vi "Test My JKI State Machine API.vi"() -> ()   [LabVIEW 2017, in "CSM Example echo DQMH.lvlib"]
doc: "------------- lvcsm -------------\n[CSMStates]\nItem 0 = \"Event Structure\"\nItem 1 = \"Idle\"\nItem 2 = \"Critical Error\"\nItem 3 = \"Async Message Posted\"\nItem 4 = \"Target Timeout Error\"\nItem 5 = \"Target Error\"\nItem 6 = \"Async Response\"\nItem 7 = \"Response\"\nItem 8 = \"Initialize Core Data\"\nItem 9 = \"VI Reference\"\nItem 10 = \"Error Handler\"\nItem 11 = \"Exit\"\nItem 12 = \"Data: Initialize\"\nItem 13 = \"Data: Cleanup\"\nItem 14 = \"UI: Initialize\"\nItem 15 = \"UI: Cursor Set\"\nItem 16 = \"UI: Front Panel State\"\nItem 17 = \"Macro: Initialize\"\nItem 18 = \"Macro: Exit\"\nItem 19 = \"New Category: 1\"\nItem 20 = \"New Category: 2\"\nItem 21 = \"Module: Start Module\"\n\n[CSMStatus]"
uses:
  CSM Example echo DQMH.lvlib
  user.lib/_NEVSTOP/Communicable State Machine(CSM)/_Support/Common/Format Timestamp.vi
  user.lib/_NEVSTOP/Communicable State Machine(CSM)/_Polymophic/Build No-Reply Asynchronous Message with Arguments.vi
  user.lib/_NEVSTOP/Communicable State Machine(CSM)/Communicable State Machine.lvlib
panel:
  out "Active Module":string[](array[string])
  in  "Select  Module":string(combo)
  out "Reply":string
  in  "X":dbl=1.0
  in  "wait for reply":bool=TRUE
  out "Reply Payload":dbl
  in  "Stop Module":bool
  in  "Start Module":bool
  in  "Test Do Something Else and Wait for Reply":bool
  in  "Hide Module Panel":bool
  in  "Show Module Panel":bool
  in  "Test Do Something Else":bool
  in  "Test Do Something":bool
  # "1. Support both Singleton and Cloneable , compare with DQMH Template\n2. Use the reply method -> as the replacement of status report in DQMH Template"
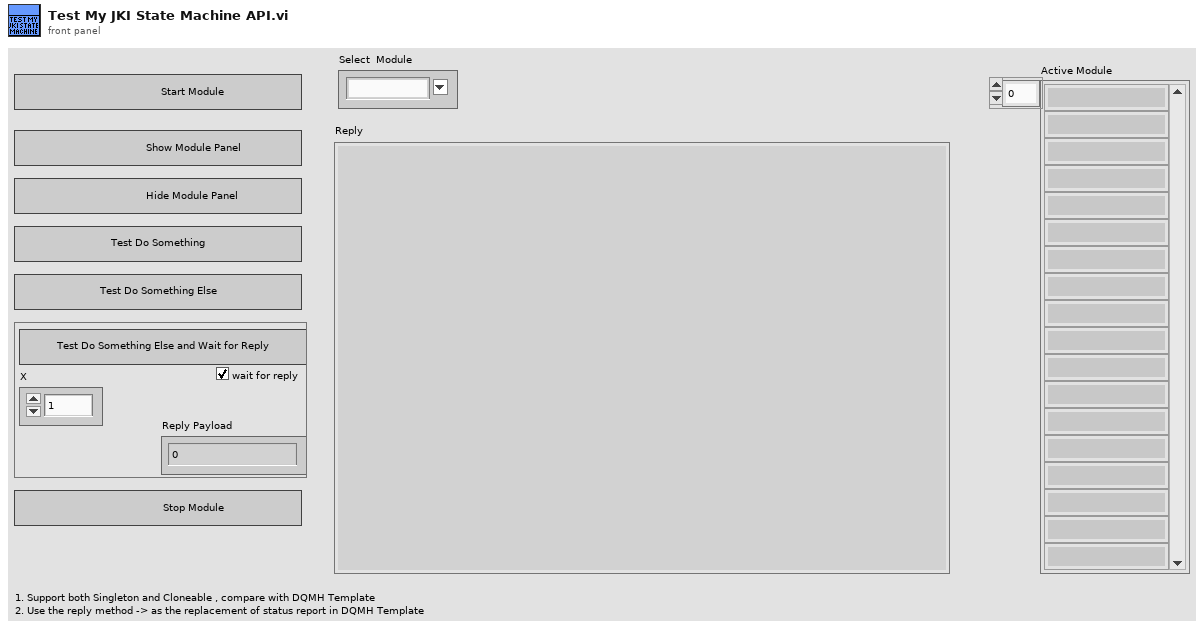
[diagram p1: front panel]
types:
  T1 = enum32{"Invalid", "Standard", "Closed", "Hidden", "Minimized", "Maximized"}
  T2 = enum32{"invalid app kind", "Development System", "Run Time System", "Student Edition", "Embedded LabVIEW", "Evaluation", "Custom"}
  T3 = typedef "Communicable State Machine.lvlib/_CSM_Response Source Message.ctl" = cluster{"‘State":string, "’Arguments":string, "’Error":errorcluster}
  T4 = cluster{"Core":cluster{"Current VI Reference":refnum<vi>, "Close Panel on Exit?":bool}, "Your Boolean data":bool, "Your string data":string, "Select  Module":refnum<vi>}
  T5 = cluster{"Current VI Reference":refnum<vi>, "Close Panel on Exit?":bool}
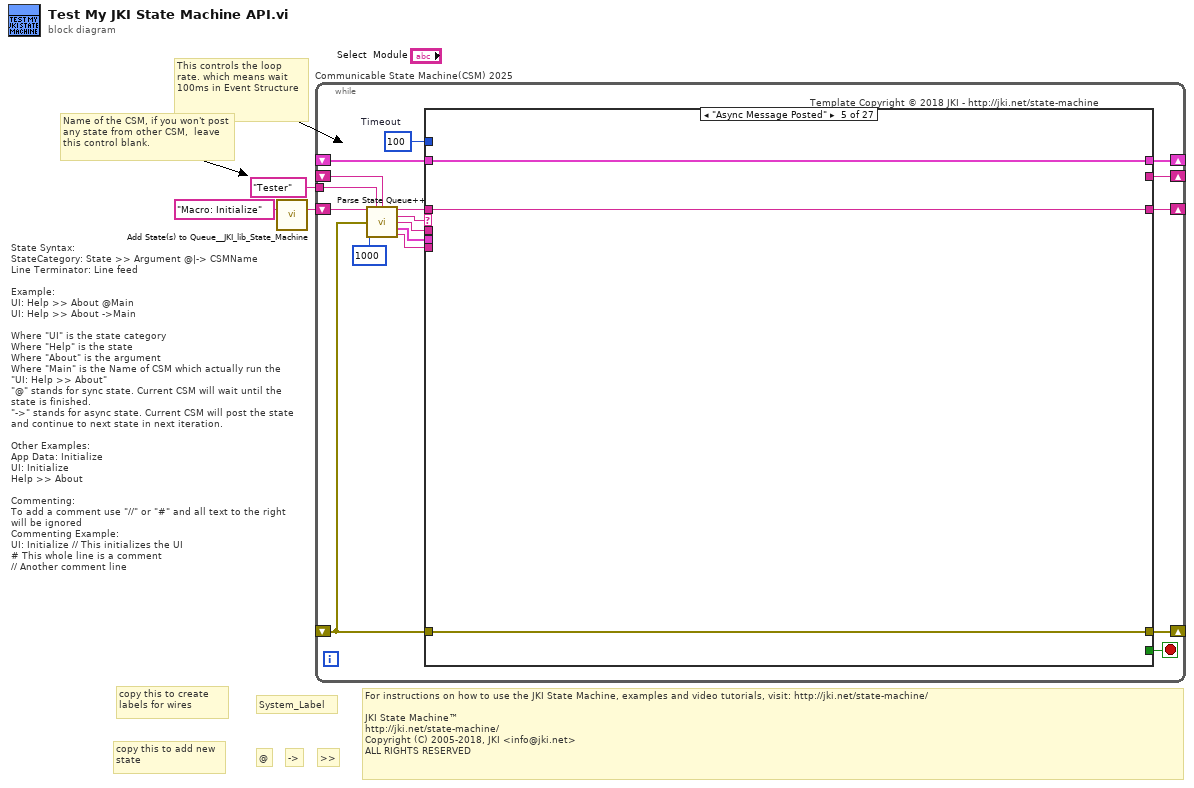
[diagram p0: block diagram]
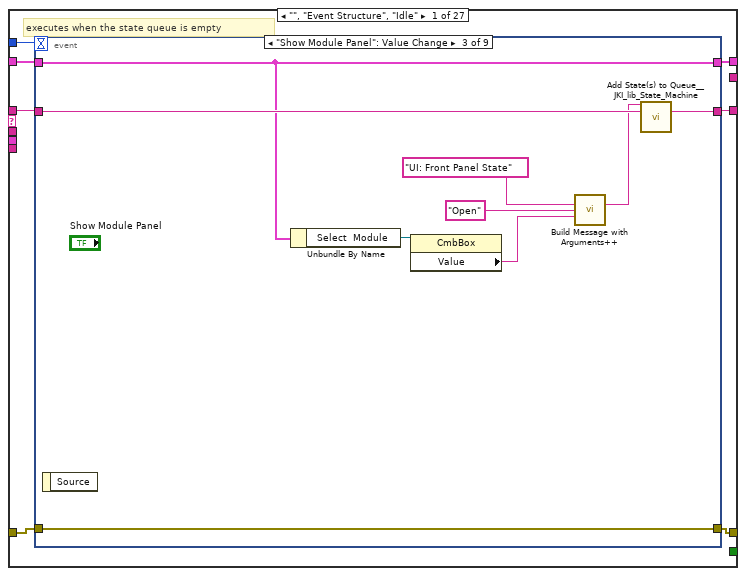
[diagram p2: hidden frame]
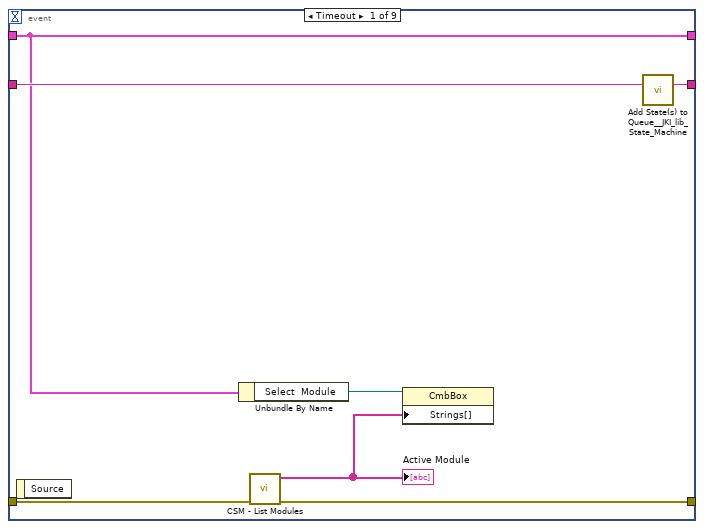
[diagram p3: hidden frame]
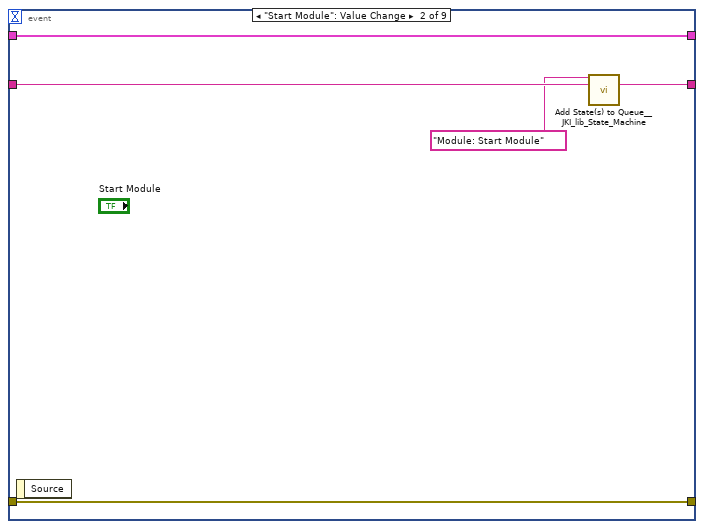
[diagram p4: hidden frame]
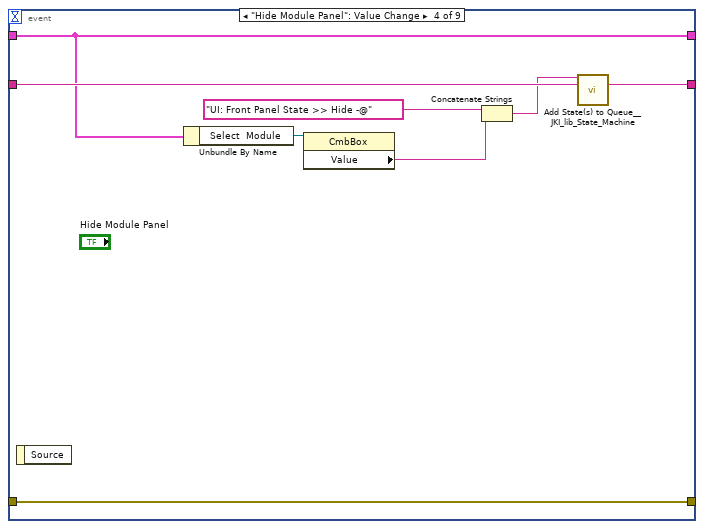
[diagram p5: hidden frame]
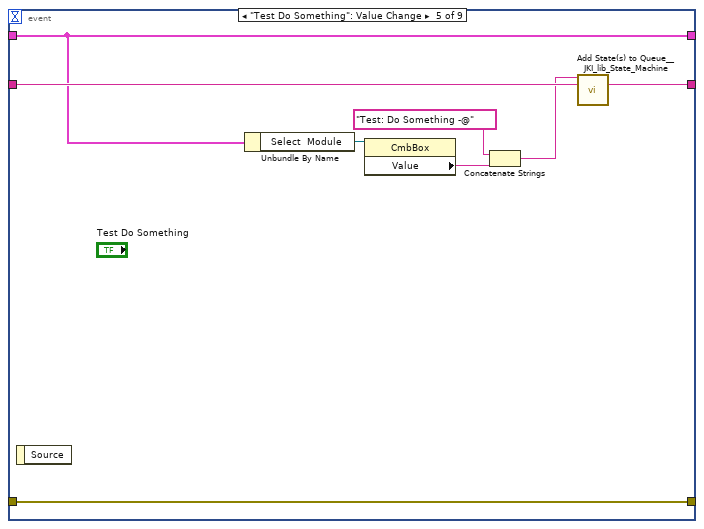
[diagram p6: hidden frame]
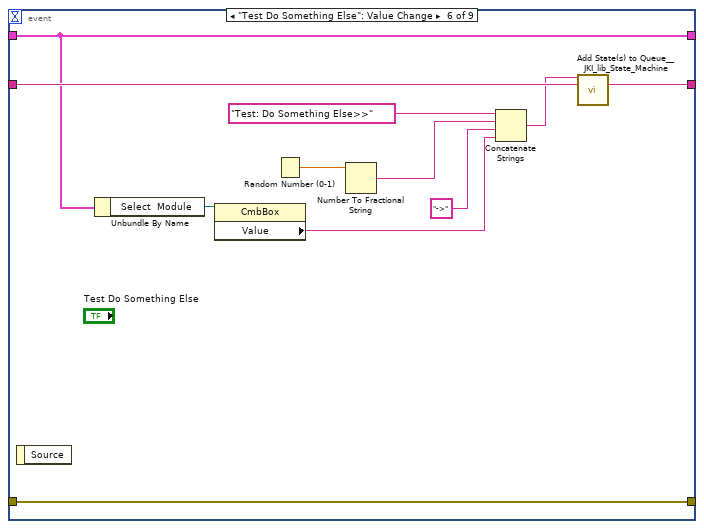
[diagram p7: hidden frame]
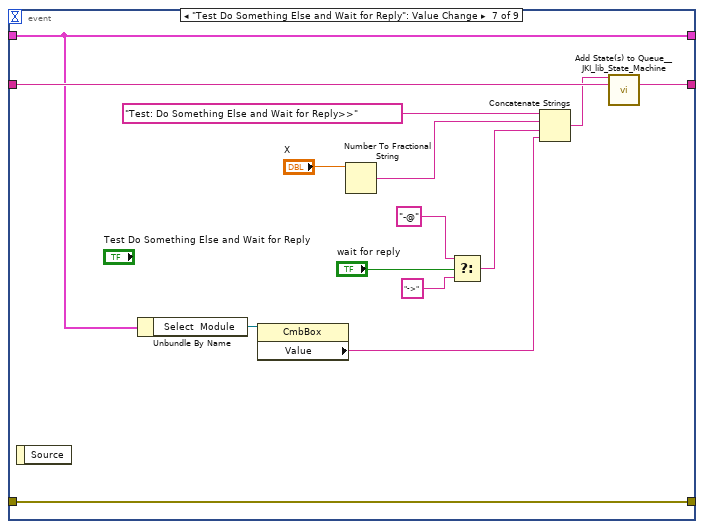
[diagram p8: hidden frame]
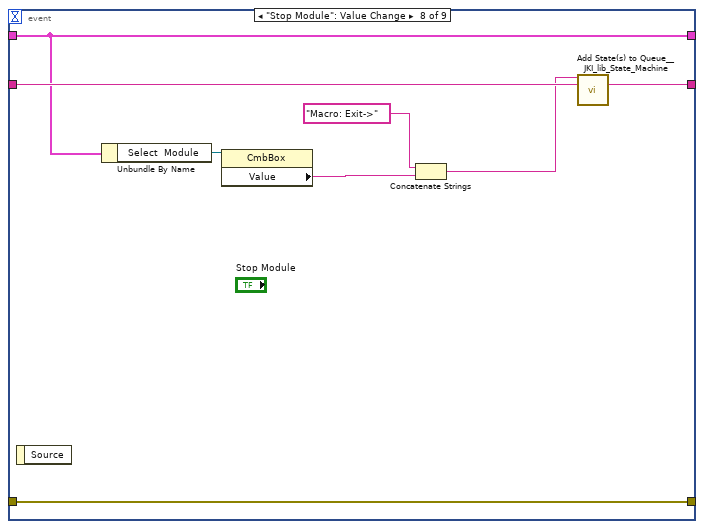
[diagram p9: hidden frame]
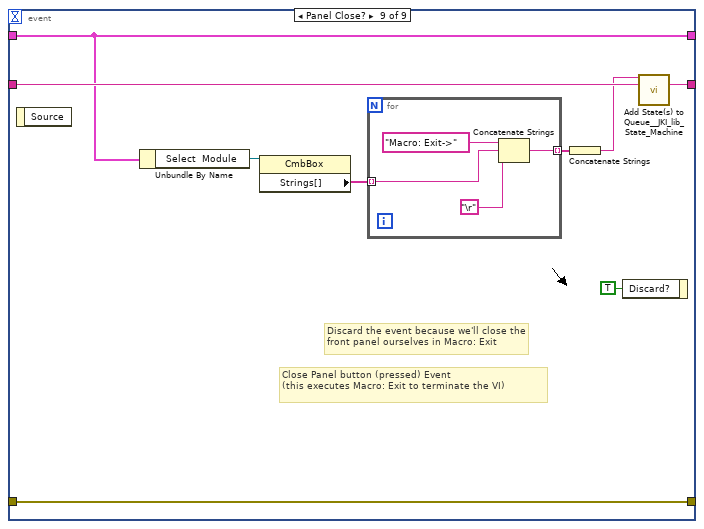
[diagram p10: hidden frame]
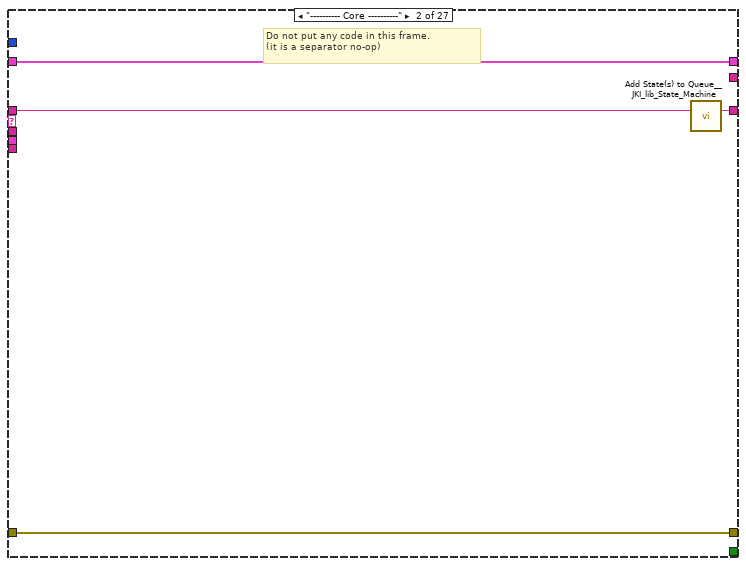
[diagram p11: hidden frame]
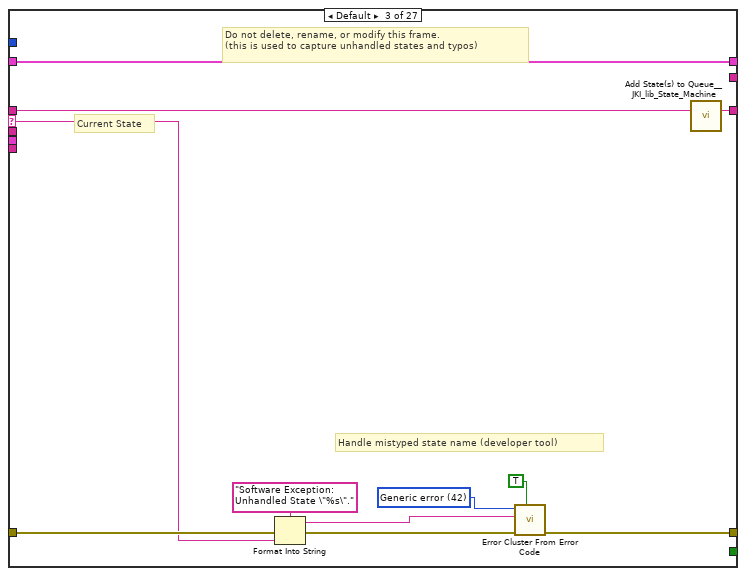
[diagram p12: hidden frame]
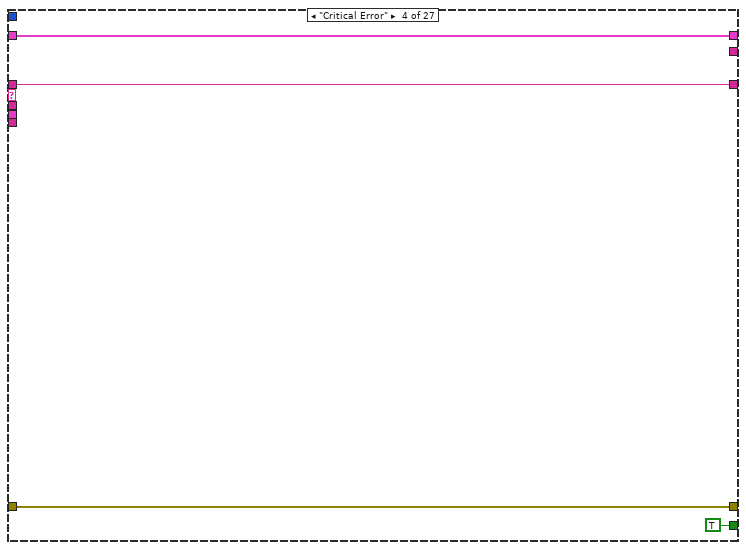
[diagram p13: hidden frame]
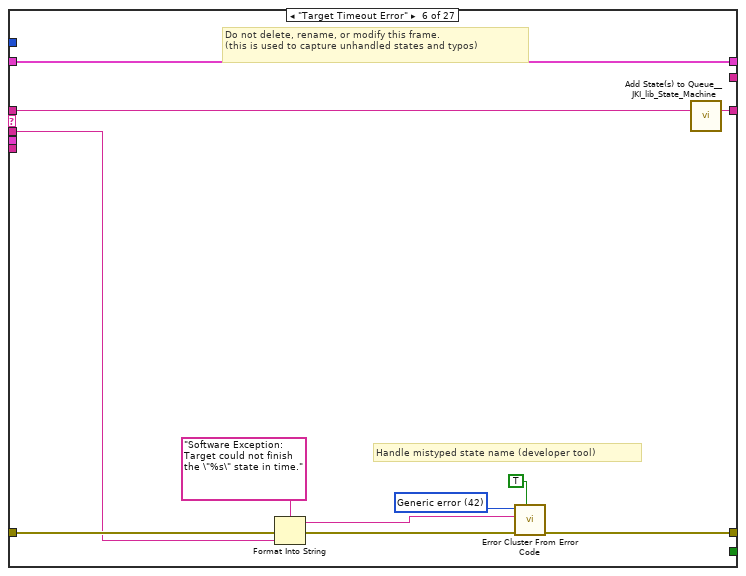
[diagram p14: hidden frame]
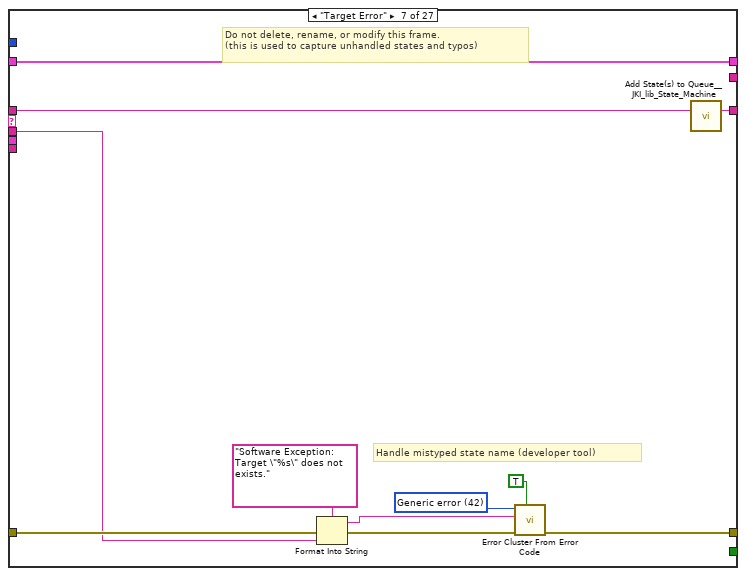
[diagram p15: hidden frame]
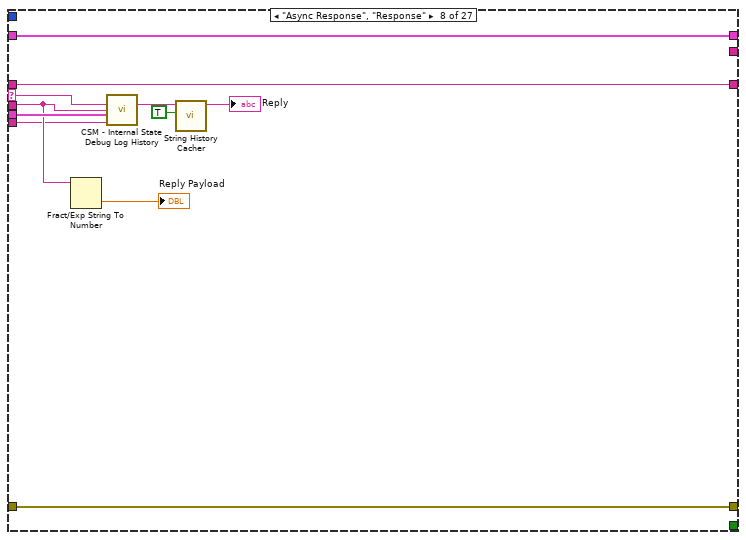
[diagram p16: hidden frame]
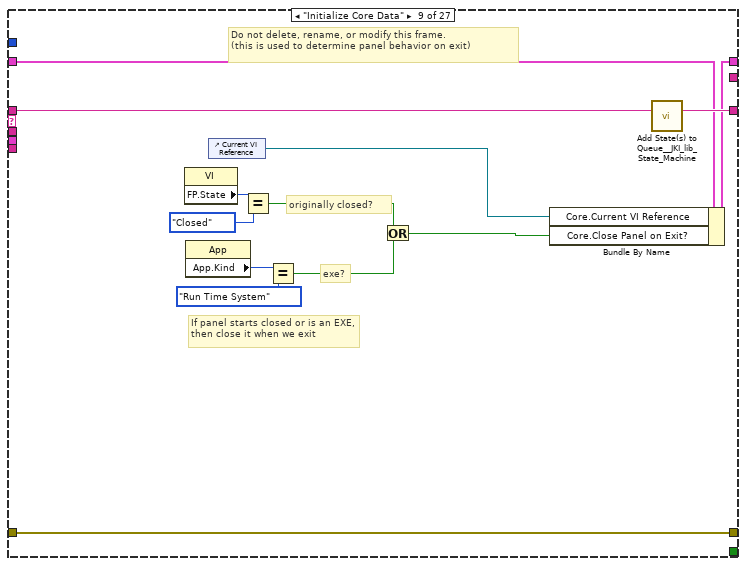
[diagram p17: hidden frame]
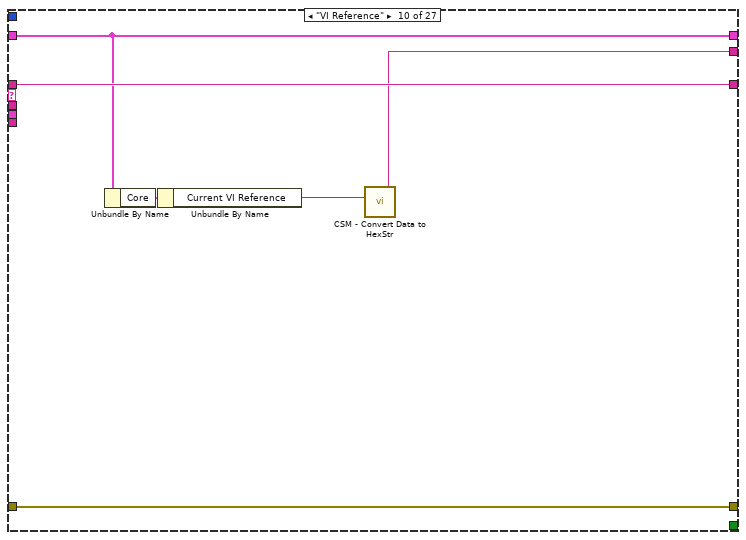
[diagram p18: hidden frame]
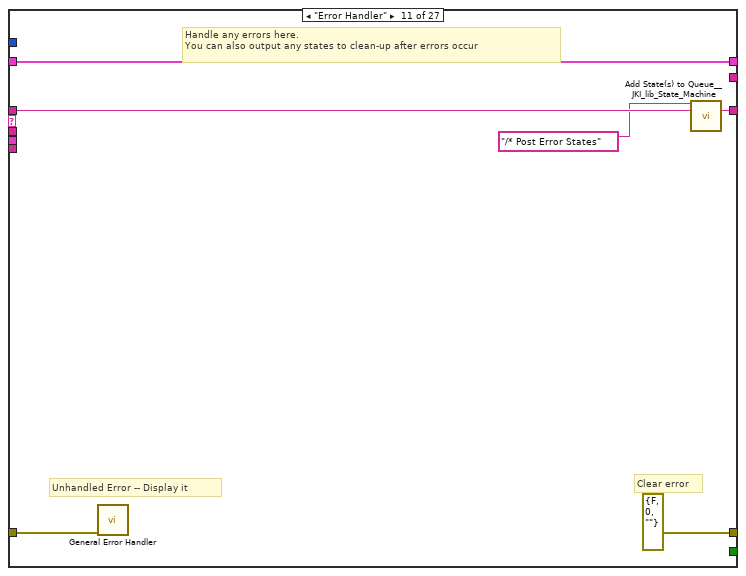
[diagram p19: hidden frame]
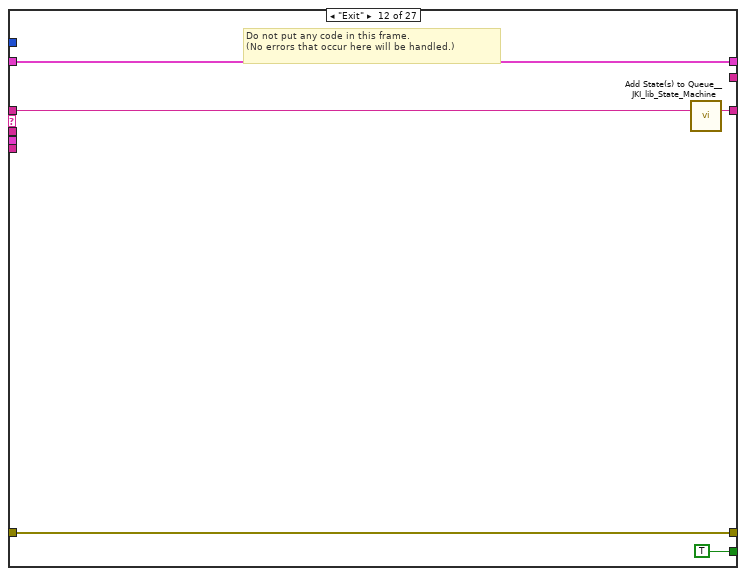
[diagram p20: hidden frame]
diagram:
  # "copy this to add new state"
  # ">>"
  # "->"
  # "@"
  # "Name of the CSM, if you won't post any state from other CSM,  leave this control blank."
  # "For instructions on how to use the JKI State Machine, examples and video tutorials, visit: http://jki.net/state-machine/\n\nJKI State Machine™\nhttp://jki.net/state-machine/\nCopyright (C) 2005-2018, JKI <info@jki.net>\nALL RIGHTS RESERVED"
  # "State Syntax:\nStateCategory: State >> Argument @|-> CSMName\nLine Terminator: Line feed\n\nExample:\nUI: Help >> About @Main\nUI: Help >> About ->Main\n\nWhere \"UI\" is the state category\nWhere \"Help\" is the state\nWhere \"About\" is the argument\nWhere \"Main\" is the Name of CSM which actually run the \"UI: Help >> About\"\n\"@\" stands for sync state. Current CSM will wait until the state is finished.\n\"->\" stands for async state. Current CSM will post the state and continue to next state in next iteration.\n\nOther Examples:\nApp Data: Initialize\nUI: Initialize\nHelp >> About\n\nCommenting:\nTo add a comment use \"//\" or \"#\" and all text to the right will be ignored\nCommenting Example:\nUI: Initialize // This initializes the UI\n# This whole line is a comment\n// Another comment line"
  # "copy this to create labels for wires"
  # "This controls the loop rate. which means wait 100ms in Event Structure"
  # "System_Label"
  n1 = call <vilib>:"Add State(s) to Queue__JKI_lib_State_Machine.vi"("State(s) in (\"\")"="Macro: Initialize") -> ("States Out"=w3:string)  [unwired: 14 in]
  n2 = while "Communicable State Machine(CSM) 2025" {
    shift-right: [w15] -> _
    shift-left: _ -> [w14]
    shift-right: [w18] -> _
    shift-left: _ -> [w12]
    shift-right: [w17] -> _
    shift-left: w3 -> [w19]
    tunnel: "Tester" ("Name(\"\" to use uuid)") -> [w8]
    shift-right: [w4] -> _
    shift-left: _ -> [w5]
    stop <- w16 stop-if-true
    w13 = 100  # Timeout
    # "Template Copyright © 2018 JKI - http://jki.net/state-machine"
    n3 = call "Parse State Queue++.vi"("State Queue"=w19, "Name (\"\" to Use UUID)"=w8, "Response Arguments"=w5, "Previous Error"=w12, "Response Timeout (-2 Use Global Settings)"=1000 ("Response Timeout(1000ms)")) -> ("Remaining States"=w20:string, "Current State"=w11:string, "Arguments"=w10:string, ">> Response Source Message >>"=w6:T3, ">> Source CSM >>"=w9:string)  [unwired: 5 in, 1 out]
    n4 = case shown="\"Async Message Posted\"" w11 {
      selector: w11 -> [_ _ w115 _ _ _ _ w162 _ _ _ _ _ _ _ _ _ _ _ _ _ _ _ _ _ _ _]
      tunnel: w20 -> [w27 w114 w119 w128 w131 w137 w148 w164 w178 w183 w190 w195 w199 w207 w213 w217 w221 w227 w238 w307 w312 w322 w326 w330 w334 w336 w345]
      tunnel: w10 -> [_ _ _ _ _ w133 w144 w158 _ _ _ _ _ _ _ _ _ w222 w232 _ _ _ _ _ _ _ _]
      tunnel: w14 -> [w25 w111 w117 w127 w130 w135 w146 w163 w171 w182 w187 w193 w196 _ w208 w214 w219 w225 w234 w304 w309 w319 w323 w327 w331 w335 w356]
      tunnel: [w24 w112 w121 w129 w132 w139 w150 w165 w175 w184 errorcluster {"status"=FALSE, "code"=0, "source"=""} ("error out") w192 w197 w204 w209 w215 w218 w223 w235 w305 w310 w320 w324 w328 w332 w337 w344] -> w18
      tunnel: w12 -> [w23 w112 w120 w129 w132 w138 w149 w165 w175 w184 w186 w192 w197 w204 w210 w215 w218 w224 w236 w305 w310 w320 w324 w328 w332 w337 w354]
      tunnel: [w26 w113 w118 w128 w131 w136 w147 w164 w177 w183 w189 w194 w198 w206 w212 w216 w220 w226 w237 w306 w311 w321 w325 w329 w333 w336 w345] -> w17
      tunnel: [_ _ _ TRUE _ _ _ _ _ _ _ TRUE _ _ _ _ _ _ _ _ _ _ _ _ _ _ _] -> w16
      tunnel: [w22 w111 w117 w127 w130 w135 w146 w163 w176 w182 w187 w193 w196 w205 w208 w214 w219 w225 w234 w304 w309 w319 w323 w327 w331 w335 w356] -> w15
      tunnel: w13 -> [w21 _ _ _ _ _ _ _ _ _ _ _ _ _ _ _ _ _ _ _ _ _ _ _ _ _ _]
      tunnel: w9 -> [_ _ _ _ _ _ _ w156 _ _ _ _ _ _ _ _ _ _ _ _ _ _ _ _ _ _ _]
      tunnel: w6 -> [_ _ _ _ _ _ _ w161 _ _ _ _ _ _ _ _ _ _ _ _ _ _ _ _ _ _ _]
      tunnel: [_ _ _ _ _ _ _ _ _ w179 _ _ _ _ _ _ _ _ _ _ _ _ _ _ _ _ w338] -> w4
      frame "", "Event Structure", "Idle" {
        # "executes when the state queue is empty"
        n5 = event shown="[2] \"Show Module Panel\": Value Change" {
          selector: _ -> [_ _ _ _ _ _ _ _ _]
          dyn-events: _ -> [_ _ _ _ _ _ _ _ _]
          timeout: w21 -> [_ _ _ _ _ _ _ _ _]
          tunnel: w27 -> [w34 w38 w48 w56 w64 w75 w89 w97 w106]
          tunnel: [w33 w37 w47 w55 w63 w74 w88 w96 w105] -> w26
          tunnel: w25 -> [w29 w39 w45 w52 w60 w66 w77 w93 w101]
          tunnel: [w31 w36 w46 w54 w62 w73 w87 w95 w104] -> w24
          tunnel: w23 -> [w32 w36 w46 w54 w62 w73 w87 w95 w104]
          tunnel: [w29 w39 w45 w52 w60 w66 w77 w93 w101] -> w22
          event Timeout {
            n6 = event-data() -> ()  [unwired: 1 in, 1 out]
            n7 = Unbundle By Name(w29) -> ("Select  Module"=w28:refnum<vi>)
            n8 = call "CSM - List Modules.vi"("Error In"=w32) -> ("error out"=w31:errorcluster, "Module Names"=w30:string[])  [unwired: 9 in]
            "Active Module" <- w30
            n9 = property class="CmbBox"(reference=w28, "Strings[]"=w30) -> ()  [unwired: 1 in, 2 out]
            n10 = call <vilib>:"Add State(s) to Queue__JKI_lib_State_Machine.vi"("State(s) in (\"\")"=w34) -> ("States Out"=w33:string)  [unwired: 14 in]
          }
          event "Start Module": Value Change {
            n11 = event-data() -> ()  [unwired: 1 in, 1 out]
            n12 = call <vilib>:"Add State(s) to Queue__JKI_lib_State_Machine.vi"("State(s) in Front (\"\")"="Module: Start Module" ("State(s) in Front (\"\")"), "State(s) in (\"\")"=w38) -> ("States Out"=w37:string)  [unwired: 13 in]
          }
          event "Show Module Panel": Value Change {
            n13 = event-data() -> ()  [unwired: 1 in, 1 out]
            n14 = Unbundle By Name(w45) -> ("Select  Module"=w44:refnum<vi>)
            n15 = property class="CmbBox"(reference=w44) -> ("Value"=w43:string)  [unwired: 1 in, 2 out]
            n16 = call-poly "Build Message with Arguments++.vi"("State With Arguments"="UI: Front Panel State" ("State(s) in Front (\"\")"), "Arguments (\"\")"="Open" ("Arguments (\"\")"), "Target Module (\"\")"=w43) -> ("CSM Message String"=w40:string)  [unwired: 12 in]
            n17 = call <vilib>:"Add State(s) to Queue__JKI_lib_State_Machine.vi"("State(s) in Front (\"\")"=w40, "State(s) in (\"\")"=w48) -> ("States Out"=w47:string)  [unwired: 13 in]
          }
          event "Hide Module Panel": Value Change {
            n18 = event-data() -> ()  [unwired: 1 in, 1 out]
            n19 = Unbundle By Name(w52) -> ("Select  Module"=w53:refnum<vi>)
            n20 = property class="CmbBox"(reference=w53) -> ("Value"=w50:string)  [unwired: 1 in, 2 out]
            n21 = Concatenate Strings("UI: Front Panel State >> Hide -@" ("State(s) in Front (\"\")"), w50) -> (w49:string)
            n22 = call <vilib>:"Add State(s) to Queue__JKI_lib_State_Machine.vi"("State(s) in Front (\"\")"=w49, "State(s) in (\"\")"=w56) -> ("States Out"=w55:string)  [unwired: 13 in]
          }
          event "Test Do Something": Value Change {
            n23 = event-data() -> ()  [unwired: 1 in, 1 out]
            n24 = Unbundle By Name(w60) -> ("Select  Module"=w61:refnum<vi>)
            n25 = property class="CmbBox"(reference=w61) -> ("Value"=w59:string)  [unwired: 1 in, 2 out]
            n26 = Concatenate Strings("Test: Do Something -@" ("State(s) in Front (\"\")"), w59) -> (w57:string)
            n27 = call <vilib>:"Add State(s) to Queue__JKI_lib_State_Machine.vi"("State(s) in Front (\"\")"=w57, "State(s) in (\"\")"=w64) -> ("States Out"=w63:string)  [unwired: 13 in]
          }
          event "Test Do Something Else": Value Change {
            n28 = event-data() -> ()  [unwired: 1 in, 1 out]
            n29 = Unbundle By Name(w66) -> ("Select  Module"=w67:refnum<vi>)
            n30 = property class="CmbBox"(reference=w67) -> ("Value"=w65:string)  [unwired: 1 in, 2 out]
            n31 = Random Number (0-1)() -> (number: 0 to 1=w72:dbl)
            n32 = Number To Fractional String(number=w72) -> (F-format string=w70:string)  [unwired: 3 in]
            n33 = Concatenate Strings("Test: Do Something Else>>" ("State(s) in Front (\"\")"), w70, "->" ("string"), w65) -> (w68:string)
            n34 = call <vilib>:"Add State(s) to Queue__JKI_lib_State_Machine.vi"("State(s) in Front (\"\")"=w68, "State(s) in (\"\")"=w75) -> ("States Out"=w74:string)  [unwired: 13 in]
          }
          event "Test Do Something Else and Wait for Reply": Value Change {
            n35 = event-data() -> ()  [unwired: 1 in, 1 out]
            n36 = Unbundle By Name(w77) -> ("Select  Module"=w78:refnum<vi>)
            n37 = property class="CmbBox"(reference=w78) -> ("Value"=w76:string)  [unwired: 1 in, 2 out]
            n38 = Number To Fractional String(number="X") -> (F-format string=w85:string)  [unwired: 3 in]
            n39 = Select(t="-@" ("string"), s="wait for reply", f="->" ("string")) -> (s? t:f=w80:string)
            n40 = Concatenate Strings("Test: Do Something Else and Wait for Reply>>" ("State(s) in Front (\"\")"), w85, w80, w76) -> (w84:string)
            n41 = call <vilib>:"Add State(s) to Queue__JKI_lib_State_Machine.vi"("State(s) in Front (\"\")"=w84, "State(s) in (\"\")"=w89) -> ("States Out"=w88:string)  [unwired: 13 in]
          }
          event "Stop Module": Value Change {
            n42 = event-data() -> ()  [unwired: 1 in, 1 out]
            n43 = Unbundle By Name(w93) -> ("Select  Module"=w94:refnum<vi>)
            n44 = property class="CmbBox"(reference=w94) -> ("Value"=w92:string)  [unwired: 1 in, 2 out]
            n45 = Concatenate Strings("Macro: Exit->" ("State(s) in Front (\"\")"), w92) -> (w90:string)
            n46 = call <vilib>:"Add State(s) to Queue__JKI_lib_State_Machine.vi"("State(s) in Front (\"\")"=w90, "State(s) in (\"\")"=w97) -> ("States Out"=w96:string)  [unwired: 13 in]
          }
          event Panel Close? {
            # "Discard the event because we'll close the front panel ourselves in Macro: Exit"
            # "Close Panel button (pressed) Event\n(this executes Macro: Exit to terminate the VI)"
            n47 = event-data() -> ()  [unwired: 1 in, 1 out]
            n48 = Unbundle By Name(w101) -> ("Select  Module"=w102:refnum<vi>)
            n49 = property class="CmbBox"(reference=w102) -> ("Strings[]"=w100:string[])  [unwired: 1 in, 2 out]
            n50 = for {
              tunnel: w100 -> [w109] mode=indexing
              tunnel: [w108] -> w99 mode=indexing
              n51 = Concatenate Strings("Macro: Exit->", w109, "\r") -> (w108:string)
            }
            n52 = Concatenate Strings(w99) -> (w98:string)
            n53 = event-data("Discard?"=TRUE) -> ()  [unwired: 1 in, 1 out]
            n54 = call <vilib>:"Add State(s) to Queue__JKI_lib_State_Machine.vi"("State(s) in Front (\"\")"=w98, "State(s) in (\"\")"=w106) -> ("States Out"=w105:string)  [unwired: 13 in]
          }
        }
      }
      frame "---------- Core ----------" {
        # "Do not put any code in this frame.\n(it is a separator no-op)"
        n55 = call <vilib>:"Add State(s) to Queue__JKI_lib_State_Machine.vi"("State(s) in (\"\")"=w114) -> ("States Out"=w113:string)  [unwired: 14 in]
      }
      frame Default {
        w124 = 42 items=["No error", "Argument error", "Memory is full", "Out of zone", "End of file", "File already open", "Generic file I/O error", "File not found", "File permission error", "Disk is full", "Duplicate path", "Too many files open", "System feature not enabled", "Resource file not found", "Cannot add resource", "Resource not found", "Image not found", "Image memory error", "Pen does not exist", "Config type invalid", "Config token not found", "Config parse error", "Config memory error", "Bad external code format", "Bad external code offset", "External code not present", "Null window", "Destroy window error", "Null menu", "Print aborted", "Bad print record", "Print driver error", "Windows error during printing", "Memory error during printing", "Print dialog error", "Generic print error", "Invalid device refnum", "Device not found", "Device parameter error", "Device unit error", "Cannot open device", "Device call aborted", "Generic error", "Cancelled by user", "Object ID too low", "Object ID too high", "Object not in heap", "Unknown heap", "Unknown object (invalid DefProc)", "Unknown object (DefProc not in table)", "Message out of range", "Invalid (null) method", "Unknown message", "Manager call not supported", "Bad address", "Network operation in progress", "Network operation timed out", "Connection is busy", "Network attribute not supported", "Network error", "Address in use", "System out of memory", "Connection aborted", "Connection refused", "Not connected", "Already connected", "Connection closed", "Initialization error (interapplication manager)", "Bad occurrence", "Wait on unbound occurrence handler", "Occurrence queue overflow", "Datalog type conflict", "Unused", "Unrecognized type (interapplication manager)", "Memory corrupt", "Failed to make temporary DLL", "Old CIN version", "Drag socket not found", "Failed to load drop-object", "Failed to register OLE object", "Failed to release OLE object", "Format specifier type mismatch", "Unknown format specifier", "Too few format specifiers", "Too many format specifiers", "Scan failed", "Newer CIN version", "Error converting to variant", "Runtime menu error", "Password tampered", "Variant attribute not found", "Incompatible variant data type", "Event data is not available", "Event Store is not present", "Occurrence is not found", "Event Queue is not created", "Event info is not available", "Refnum passed is NULL", "Error retrieving Class GUID", "Error retrieving CoClass GUID", "Error retrieving TypeLib GUID.", "Bad built application magic bytes.", "Specific driver is different from the specific driver associated with the Logical Name.", "There is no session opened to the class driver.", "Max Error", "MAX - Error with config objects", "MAX - Error loading configuration", "MAX - Group not supported"]
        # "Current State"
        # "Do not delete, rename, or modify this frame.\n(this is used to capture unhandled states and typos)"
        # "Handle mistyped state name (developer tool)"
        n56 = Format Into String(format string="Software Exception: Unhandled State \"%s\"." ("message"), error in=w120, w115) -> (resulting string=w123:string, error out=w122:errorcluster)  [unwired: 1 in]
        n57 = call <vilib>:"Error Cluster From Error Code.vi"("show call chain? (False)"=TRUE, "error in (no error)"=w122, "error message (\"\")"=w123, "error code (0)"=w124) -> ("error out"=w121:errorcluster)  [unwired: 5 in]
        n58 = call <vilib>:"Add State(s) to Queue__JKI_lib_State_Machine.vi"("State(s) in (\"\")"=w119) -> ("States Out"=w118:string)  [unwired: 14 in]
      }
      frame "Critical Error" {
      }
      frame "Async Message Posted" {
      }
      frame "Target Timeout Error" {
        w142 = 42 items=["No error", "Argument error", "Memory is full", "Out of zone", "End of file", "File already open", "Generic file I/O error", "File not found", "File permission error", "Disk is full", "Duplicate path", "Too many files open", "System feature not enabled", "Resource file not found", "Cannot add resource", "Resource not found", "Image not found", "Image memory error", "Pen does not exist", "Config type invalid", "Config token not found", "Config parse error", "Config memory error", "Bad external code format", "Bad external code offset", "External code not present", "Null window", "Destroy window error", "Null menu", "Print aborted", "Bad print record", "Print driver error", "Windows error during printing", "Memory error during printing", "Print dialog error", "Generic print error", "Invalid device refnum", "Device not found", "Device parameter error", "Device unit error", "Cannot open device", "Device call aborted", "Generic error", "Cancelled by user", "Object ID too low", "Object ID too high", "Object not in heap", "Unknown heap", "Unknown object (invalid DefProc)", "Unknown object (DefProc not in table)", "Message out of range", "Invalid (null) method", "Unknown message", "Manager call not supported", "Bad address", "Network operation in progress", "Network operation timed out", "Connection is busy", "Network attribute not supported", "Network error", "Address in use", "System out of memory", "Connection aborted", "Connection refused", "Not connected", "Already connected", "Connection closed", "Initialization error (interapplication manager)", "Bad occurrence", "Wait on unbound occurrence handler", "Occurrence queue overflow", "Datalog type conflict", "Unused", "Unrecognized type (interapplication manager)", "Memory corrupt", "Failed to make temporary DLL", "Old CIN version", "Drag socket not found", "Failed to load drop-object", "Failed to register OLE object", "Failed to release OLE object", "Format specifier type mismatch", "Unknown format specifier", "Too few format specifiers", "Too many format specifiers", "Scan failed", "Newer CIN version", "Error converting to variant", "Runtime menu error", "Password tampered", "Variant attribute not found", "Incompatible variant data type", "Event data is not available", "Event Store is not present", "Occurrence is not found", "Event Queue is not created", "Event info is not available", "Refnum passed is NULL", "Error retrieving Class GUID", "Error retrieving CoClass GUID", "Error retrieving TypeLib GUID.", "Bad built application magic bytes.", "Specific driver is different from the specific driver associated with the Logical Name.", "There is no session opened to the class driver.", "Max Error", "MAX - Error with config objects", "MAX - Error loading configuration", "MAX - Group not supported"]
        # "Do not delete, rename, or modify this frame.\n(this is used to capture unhandled states and typos)"
        # "Handle mistyped state name (developer tool)"
        n59 = Format Into String(format string="Software Exception: Target could not finish the \"%s\" state in time." ("message"), error in=w138, w133) -> (resulting string=w141:string, error out=w140:errorcluster)  [unwired: 1 in]
        n60 = call <vilib>:"Error Cluster From Error Code.vi"("show call chain? (False)"=TRUE, "error in (no error)"=w140, "error message (\"\")"=w141, "error code (0)"=w142) -> ("error out"=w139:errorcluster)  [unwired: 5 in]
        n61 = call <vilib>:"Add State(s) to Queue__JKI_lib_State_Machine.vi"("State(s) in (\"\")"=w137) -> ("States Out"=w136:string)  [unwired: 14 in]
      }
      frame "Target Error" {
        w153 = 42 items=["No error", "Argument error", "Memory is full", "Out of zone", "End of file", "File already open", "Generic file I/O error", "File not found", "File permission error", "Disk is full", "Duplicate path", "Too many files open", "System feature not enabled", "Resource file not found", "Cannot add resource", "Resource not found", "Image not found", "Image memory error", "Pen does not exist", "Config type invalid", "Config token not found", "Config parse error", "Config memory error", "Bad external code format", "Bad external code offset", "External code not present", "Null window", "Destroy window error", "Null menu", "Print aborted", "Bad print record", "Print driver error", "Windows error during printing", "Memory error during printing", "Print dialog error", "Generic print error", "Invalid device refnum", "Device not found", "Device parameter error", "Device unit error", "Cannot open device", "Device call aborted", "Generic error", "Cancelled by user", "Object ID too low", "Object ID too high", "Object not in heap", "Unknown heap", "Unknown object (invalid DefProc)", "Unknown object (DefProc not in table)", "Message out of range", "Invalid (null) method", "Unknown message", "Manager call not supported", "Bad address", "Network operation in progress", "Network operation timed out", "Connection is busy", "Network attribute not supported", "Network error", "Address in use", "System out of memory", "Connection aborted", "Connection refused", "Not connected", "Already connected", "Connection closed", "Initialization error (interapplication manager)", "Bad occurrence", "Wait on unbound occurrence handler", "Occurrence queue overflow", "Datalog type conflict", "Unused", "Unrecognized type (interapplication manager)", "Memory corrupt", "Failed to make temporary DLL", "Old CIN version", "Drag socket not found", "Failed to load drop-object", "Failed to register OLE object", "Failed to release OLE object", "Format specifier type mismatch", "Unknown format specifier", "Too few format specifiers", "Too many format specifiers", "Scan failed", "Newer CIN version", "Error converting to variant", "Runtime menu error", "Password tampered", "Variant attribute not found", "Incompatible variant data type", "Event data is not available", "Event Store is not present", "Occurrence is not found", "Event Queue is not created", "Event info is not available", "Refnum passed is NULL", "Error retrieving Class GUID", "Error retrieving CoClass GUID", "Error retrieving TypeLib GUID.", "Bad built application magic bytes.", "Specific driver is different from the specific driver associated with the Logical Name.", "There is no session opened to the class driver.", "Max Error", "MAX - Error with config objects", "MAX - Error loading configuration", "MAX - Group not supported"]
        # "Do not delete, rename, or modify this frame.\n(this is used to capture unhandled states and typos)"
        # "Handle mistyped state name (developer tool)"
        n62 = Format Into String(format string="Software Exception: Target \"%s\" does not exists." ("message"), error in=w149, w144) -> (resulting string=w152:string, error out=w151:errorcluster)  [unwired: 1 in]
        n63 = call <vilib>:"Error Cluster From Error Code.vi"("show call chain? (False)"=TRUE, "error in (no error)"=w151, "error message (\"\")"=w152, "error code (0)"=w153) -> ("error out"=w150:errorcluster)  [unwired: 5 in]
        n64 = call <vilib>:"Add State(s) to Queue__JKI_lib_State_Machine.vi"("State(s) in (\"\")"=w148) -> ("States Out"=w147:string)  [unwired: 14 in]
      }
      frame "Async Response", "Response" {
        n65 = Fract/Exp String To Number(string=w158) -> (number=→"Reply Payload":dbl)  [unwired: 3 in, 1 out]
        n66 = call "CSM - Internal State Debug Log History.vi"("State"=w162, "Arguments (\"\")"=w158, ">> Response Source Message >>"=w161, "Source (\"\")"=w156) -> ("Debug Log"=w160:string)  [unwired: 11 in]
        n67 = call "String History Cacher.vi"("Include Timestamp? (T)"=TRUE ("Include Timestamp(F)"), "String"=w160) -> ("String Cache"=→"Reply":string)  [unwired: 9 in]
      }
      frame "Initialize Core Data" {
        # "Do not delete, rename, or modify this frame.\n(this is used to determine panel behavior on exit)"
        # "originally closed?"
        # "exe?"
        # "If panel starts closed or is an EXE, then close it when we exit"
        n68 = property class="VI"() -> ("FP.State"=w168:T1)  [unwired: 2 in, 2 out]
        n69 = property class="App"() -> ("App.Kind"=w174:T2)  [unwired: 2 in, 2 out]
        n70 = control-ref of="Current VI Reference"() -> (w169:refnum<vi>)
        n71 = Equal?(x=w168, y=T1."Closed" ("Front Panel Window:State")) -> (x = y?=w166:bool)
        n72 = Equal?(x=w174, y=T2."Run Time System" ("Application:Kind")) -> (x = y?=w172:bool)
        n73 = Or(x=w166, y=w172) -> (x .or. y?=w170:bool)
        n74 = Bundle By Name(cluster=w171, "Core.Current VI Reference"=w169, "Core.Close Panel on Exit?"=w170) -> (w176:T4)
        n75 = call <vilib>:"Add State(s) to Queue__JKI_lib_State_Machine.vi"("State(s) in (\"\")"=w178) -> ("States Out"=w177:string)  [unwired: 14 in]
      }
      frame "VI Reference" {
        n76 = Unbundle By Name(w182) -> ("Core"=w181:T5)
        n77 = Unbundle By Name(w181) -> ("Current VI Reference"=w180:refnum<vi>)
        n78 = call "CSM - Convert Data to HexStr.vi"("Variant"=w180) -> ("HEX String (0-9,A-F)"=w179:string)  [unwired: 8 in]
      }
      frame "Error Handler" {
        # "Unhandled Error -- Display it"
        # "Handle any errors here.\nYou can also output any states to clean-up after errors occur"
        # "Clear error"
        n79 = call <vilib>:"General Error Handler.vi"("error in (no error)"=w186) -> ()  [unwired: 10 in, 5 out]
        n80 = call <vilib>:"Add State(s) to Queue__JKI_lib_State_Machine.vi"("State(s) in Front (\"\")"="/* Post Error States", "State(s) in (\"\")"=w190) -> ("States Out"=w189:string)  [unwired: 13 in]
      }
      frame "Exit" {
        # "Do not put any code in this frame.\n(No errors that occur here will be handled.)"
        n81 = call <vilib>:"Add State(s) to Queue__JKI_lib_State_Machine.vi"("State(s) in (\"\")"=w195) -> ("States Out"=w194:string)  [unwired: 14 in]
      }
      frame "---------- Data ----------" {
        # "Do not put any code in this frame.\n(It is a separator no-op. You can make a copy of this frame to create a new Data frame)"
        n82 = call <vilib>:"Add State(s) to Queue__JKI_lib_State_Machine.vi"("State(s) in (\"\")"=w199) -> ("States Out"=w198:string)  [unwired: 14 in]
      }
      frame "Data: Initialize" {
        w201 = T5 {"Current VI Reference"=refnum, "Close Panel on Exit?"=FALSE}  # Core
        w203 = TRUE  # Your Boolean data
        w202 = ""  # Your string data
        # "do not delete - used by framework"
        # "Expand Bundle to add new data elements to shift register data."
        # "Add new data here."
        # "Data names and types of shift register data are defined by this bundle."
        # "Initialize the shift-register data, here.\n(data names are defined by what you wire into the bundle function)"
        n83 = control-ref of="Select  Module"() -> (w200:refnum<vi>)
        n84 = Bundle("Core"=w201, "Your Boolean data"=w203, "Your string data"=w202, "Select  Module"=w200) -> (w205:T4)  [unwired: 1 in]
        n85 = call <vilib>:"Add State(s) to Queue__JKI_lib_State_Machine.vi"("State(s) in (\"\")"=w207) -> ("States Out"=w206:string)  [unwired: 14 in]
      }
      frame "Data: Cleanup" {
        # "Cleanup any data and references, here.\n(this is called automatically, by the Macro: Exit)"
        n86 = Unbundle By Name(w208) -> ("Core.Current VI Reference"=w211:refnum<vi>)
        n87 = Close Reference(reference=w211, error in (no error)=w210) -> (error out=w209:errorcluster)
        n88 = call <vilib>:"Add State(s) to Queue__JKI_lib_State_Machine.vi"("State(s) in (\"\")"=w213) -> ("States Out"=w212:string)  [unwired: 14 in]
      }
      frame "---------- UI ----------" {
        # "Do not put any code in this frame.\n(It is a separator no-op. You can make a copy of this frame to create a new UI frame)"
        n89 = call <vilib>:"Add State(s) to Queue__JKI_lib_State_Machine.vi"("State(s) in (\"\")"=w217) -> ("States Out"=w216:string)  [unwired: 14 in]
      }
      frame "UI: Initialize" {
        # "Initialize the User Interface, here.\n(this is called automatically, by the Macro: Init)"
        n90 = call <vilib>:"Add State(s) to Queue__JKI_lib_State_Machine.vi"("State(s) in (\"\")"=w221) -> ("States Out"=w220:string)  [unwired: 14 in]
      }
      frame "UI: Cursor Set" {
        # "Argument"
        # "Set and Unset Cursor Busy.\n(Usage: \"UI: Cursor Set >> Busy|Idle\")"
        n91 = case shown="\"Idle\", Default" w222 {
          tunnel: w224 -> [w229 w231]
          tunnel: [w228 w230] -> w223
          frame "Idle", Default {
            n92 = call <vilib>:"Unset Busy.vi"("error in (no error)"=w229) -> ("error out"=w228:errorcluster)  [unwired: 10 in]
          }
          frame "Busy" {
            n93 = call <vilib>:"Set Busy.vi"("error in (no error)"=w231) -> ("error out"=w230:errorcluster)  [unwired: 9 in, 1 out]
          }
        }
        n94 = call <vilib>:"Add State(s) to Queue__JKI_lib_State_Machine.vi"("State(s) in (\"\")"=w227) -> ("States Out"=w226:string)  [unwired: 14 in]
      }
      frame "UI: Front Panel State" {
        # "Argument"
        # "Set Front Panel Open or Closed\n(Usage: \"UI: Front Panel State >> Open|Close\")"
        n95 = Unbundle By Name(w234) -> ("Core.Current VI Reference"=w233:refnum<vi>)
        n96 = case shown="\"Hidden\", \"Hide\"" w232 {
          tunnel: w236 -> [w244 w259 w270 w283 w296]
          tunnel: [w246 w260 w272 w285 w298] -> w235
          tunnel: w233 -> [w245 w257 w271 w284 w297]
          frame "Open", "Standard", Default {
            w239 = T1."Standard" ("State")
            n97 = property class="VI"(reference=w245, error in=w244) -> (reference out=w242:refnum<vi>, error out=w243:errorcluster, "FP.State"=w241:T1)
            n98 = Not Equal?(x=w241, y=w239) -> (x != y?=w240:bool)
            n99 = case shown="True" w240 {
              tunnel: [w250 w252] -> w246
              tunnel: w243 -> [w249 w252]
              tunnel: w242 -> [w248 _]
              tunnel: w239 -> [w247 _]
              frame True {
                n100 = invoke class="VI" method="FP.Open"(reference=w248, error in=w249, "Activate"=TRUE, "State"=w247) -> (error out=w250:errorcluster)  [unwired: 1 in, 4 out]
              }
              frame False {
              }
            }
          }
          frame "Close", "Closed" {
            n101 = property class="VI"(reference=w257, error in=w259) -> (reference out=w256:refnum<vi>, error out=w258:errorcluster, "FP.State"=w254:T1)
            n102 = Not Equal?(x=w254, y=T1."Closed" ("Front Panel Window:State")) -> (x != y?=w253:bool)
            n103 = case shown="True" w253 {
              tunnel: [w261 w264] -> w260
              tunnel: w258 -> [w261 w263]
              tunnel: w256 -> [_ w262]
              frame False {
              }
              frame True {
                n104 = invoke class="VI" method="FP.Close"(reference=w262, error in=w263) -> (error out=w264:errorcluster)  [unwired: 1 in, 2 out]
              }
            }
          }
          frame "Hidden", "Hide" {
            w265 = T1."Hidden" ("State")
            n105 = property class="VI"(reference=w271, error in=w270) -> (reference out=w268:refnum<vi>, error out=w269:errorcluster, "FP.State"=w267:T1)
            n106 = Not Equal?(x=w267, y=w265) -> (x != y?=w266:bool)
            n107 = case shown="True" w266 {
              tunnel: [w276 w277] -> w272
              tunnel: w269 -> [w275 w277]
              tunnel: w268 -> [w274 _]
              tunnel: w265 -> [w273 _]
              frame True {
                n108 = invoke class="VI" method="FP.Open"(reference=w274, error in=w275, "State"=w273) -> (error out=w276:errorcluster)  [unwired: 2 in, 4 out]
              }
              frame False {
              }
            }
          }
          frame "Minimize", "Minimized" {
            w278 = T1."Minimized" ("State")
            n109 = property class="VI"(reference=w284, error in=w283) -> (reference out=w281:refnum<vi>, error out=w282:errorcluster, "FP.State"=w280:T1)
            n110 = Not Equal?(x=w280, y=w278) -> (x != y?=w279:bool)
            n111 = case shown="True" w279 {
              tunnel: [w289 w290] -> w285
              tunnel: w282 -> [w288 w290]
              tunnel: w281 -> [w287 _]
              tunnel: w278 -> [w286 _]
              frame True {
                n112 = invoke class="VI" method="FP.Open"(reference=w287, error in=w288, "State"=w286) -> (error out=w289:errorcluster)  [unwired: 2 in, 4 out]
              }
              frame False {
              }
            }
          }
          frame "Maximize", "Maximized" {
            w291 = T1."Maximized" ("State")
            n113 = property class="VI"(reference=w297, error in=w296) -> (reference out=w294:refnum<vi>, error out=w295:errorcluster, "FP.State"=w293:T1)
            n114 = Not Equal?(x=w293, y=w291) -> (x != y?=w292:bool)
            n115 = case shown="True" w292 {
              tunnel: [w302 w303] -> w298
              tunnel: w295 -> [w301 w303]
              tunnel: w294 -> [w300 _]
              tunnel: w291 -> [w299 _]
              frame True {
                n116 = invoke class="VI" method="FP.Open"(reference=w300, error in=w301, "State"=w299) -> (error out=w302:errorcluster)  [unwired: 2 in, 4 out]
              }
              frame False {
              }
            }
          }
        }
        n117 = call <vilib>:"Add State(s) to Queue__JKI_lib_State_Machine.vi"("State(s) in (\"\")"=w238) -> ("States Out"=w237:string)  [unwired: 14 in]
      }
      frame "---------- Macro ----------" {
        # "Do not put any code in this frame.\n(It is a separator no-op. You can make a copy of this frame to create a new Macro frame)"
        n118 = call <vilib>:"Add State(s) to Queue__JKI_lib_State_Machine.vi"("State(s) in (\"\")"=w307) -> ("States Out"=w306:string)  [unwired: 14 in]
      }
      frame "Macro: Initialize" {
        w308 = "Data: Initialize\nInitialize Core Data\nUI: Initialize\nUI: Front Panel State >> Open"  # Data: Initialize Initialize Core Data UI: Initialize UI: Front Panel State >> Open
        # "Initialization Macro\n(This is called once, when the VI starts)"
        n119 = call <vilib>:"Add State(s) to Queue__JKI_lib_State_Machine.vi"("State(s) in Front (\"\")"=w308, "State(s) in (\"\")"=w312) -> ("States Out"=w311:string)  [unwired: 13 in]
      }
      frame "Macro: Exit" {
        # "Exit Macro\n(This is called once, when the VI exits)"
        n120 = Unbundle By Name(w319) -> ("Core.Close Panel on Exit?"=w318:bool)
        n121 = Select(t="UI: Front Panel State >> Close", s=w318, f="") -> (s? t:f=w315:string)
        n122 = call <vilib>:"Add State(s) to Queue__JKI_lib_State_Machine.vi"("State(s) in (\"\")"=w315, "State(s) at Back (\"\")"="Data: Cleanup\nExit") -> ("States Out"=w313:string)  [unwired: 13 in]
        n123 = call <vilib>:"Add State(s) to Queue__JKI_lib_State_Machine.vi"("State(s) in Front (\"\")"=w313, "State(s) in (\"\")"=w322) -> ("States Out"=w321:string)  [unwired: 13 in]
      }
      frame "---------- New Category ----------" {
        # "Template Separator\n(You can make a copy of, or modify, this frame)"
        n124 = call <vilib>:"Add State(s) to Queue__JKI_lib_State_Machine.vi"("State(s) in (\"\")"=w326) -> ("States Out"=w325:string)  [unwired: 14 in]
      }
      frame "New Category: 1" {
        # "Your code here.\n(You can make a copy of, or modify, this frame)"
        n125 = call <vilib>:"Add State(s) to Queue__JKI_lib_State_Machine.vi"("State(s) in (\"\")"=w330) -> ("States Out"=w329:string)  [unwired: 14 in]
      }
      frame "New Category: 2" {
        # "Your code here.\n(You can make a copy of, or modify, this frame)"
        n126 = call <vilib>:"Add State(s) to Queue__JKI_lib_State_Machine.vi"("State(s) in (\"\")"=w334) -> ("States Out"=w333:string)  [unwired: 14 in]
      }
      frame "---------- Module ----------" {
      }
      frame "Module: Start Module" {
        n127 = vi-ref "My JKI State Machine Module.vi"() -> (w355:refnum<vi>)
        n128 = property class="VI"(reference=w355, error in=w354) -> (error out=w353:errorcluster, "Path"=w352:path)  [unwired: 1 out]
        n129 = feedback #1(0) -> (w342:i32)
        n130 = Increment(x=w342) -> (x+1=w341:i32)
        n131 = feedback-in #1(w341) -> ()
        n132 = Open VI Reference(type specifier VI Refnum (for type only)=refnum<vi> refnum, vi path=w352, options=128, error in (no error)=w353) -> (vi reference=w349:refnum<vi>, error out=w348:errorcluster)  [unwired: 2 in]
        n133 = Number To Decimal String(number=w341) -> (decimal integer string=w340:string)  [unwired: 1 in]
        n134 = Concatenate Strings("M" ("Module Name"), w340) -> (w338:string)
        n135 = call-by-ref "Start Asynchronous Call"(reference=w349, error in=w348, "Module Name"=w338) -> (reference out=w346:refnum<vi>, error out=w347:errorcluster)  [unwired: 11 in]
        n136 = Close Reference(reference=w346, error in (no error)=w347) -> (error out=w344:errorcluster)
      }
    }
  }
